vi "WS2812 Write N Pixels.vi"(7 "Refresh?":bool=TRUE, 8 "Error In":errorcluster, 9 "Colors":u32[](array[colorbox]), 10 "Start Pixel Index":u16, 11 "LINX Device Config":T1) -> (0 "Error Out":errorcluster, 3 "LINX Device Config":T1)   [LabVIEW 2014, in "LMH-LINX.lvlib" / "Device.lvlib"]
uses:
  <vilib>/MakerHub/LINX/Private/Device/Device.lvlib
  <vilib>/MakerHub/LINX/Private/Device/Type Defs/LINX Device Config.ctl
  <vilib>/MakerHub/LINX/Private/Type Defs/Interface.ctl
  <vilib>/MakerHub/LINX/Private/Device/Type Defs/TCP Config.ctl
  <vilib>/MakerHub/LINX/Private/Device/Type Defs/Channels.ctl
  <vilib>/MakerHub/LINX/Private/Type Defs/Error Type.ctl
  <vilib>/MakerHub/LINX/LMH-LINX.lvlib
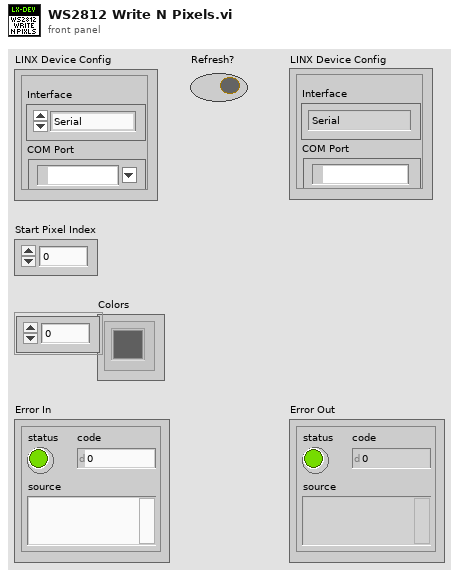
[diagram p1: front panel]
types:
  T1 = typedef "LMH-LINX.lvlib/Device.lvlib/LINX Device Config.ctl" = cluster{"Interface":T2, "COM Port":refnum<visa-resource-name>, "TCP Configuration":T3, "Device Family":u8, "Device ID":u8, "Device Name":string, "TCP Ref":refnum<k5>, "Channels":T4}
  T2 = typedef "LMH-LINX.lvlib/Interface.ctl" = enum16{"Serial", "TCP"}
  T3 = typedef "LMH-LINX.lvlib/Device.lvlib/TCP Config.ctl" = cluster{"IP Address":string, "Port":u16}
  T4 = typedef "LMH-LINX.lvlib/Channels.ctl" = cluster{"DI":u8[], "DO":u8[], "AI":u8[], "AO":u8[], "PWM":u8[], "QE":u8[], "UART":u8[], "I2C 2":u8[], "SPI":u8[], "CAN":u8[], "Servo":u8[], "AI Ref (V)":dbl, "AI Resolution (Bits)":u8, "AO Ref (V)":dbl, "AO Resolution (Bits)":u8}
  T5 = typedef "LMH-LINX.lvlib/Error Type.ctl" = enum16{"Unknown", "Timeout", "Corrupt Return Packet", "Unable To Connect", "Command Not Supported", "Channel DNE", "Invalid COM Config", "Firmware Version Mismatch", "myRIO Support", "CMD Specific Error", "Local IO Not Supported"}
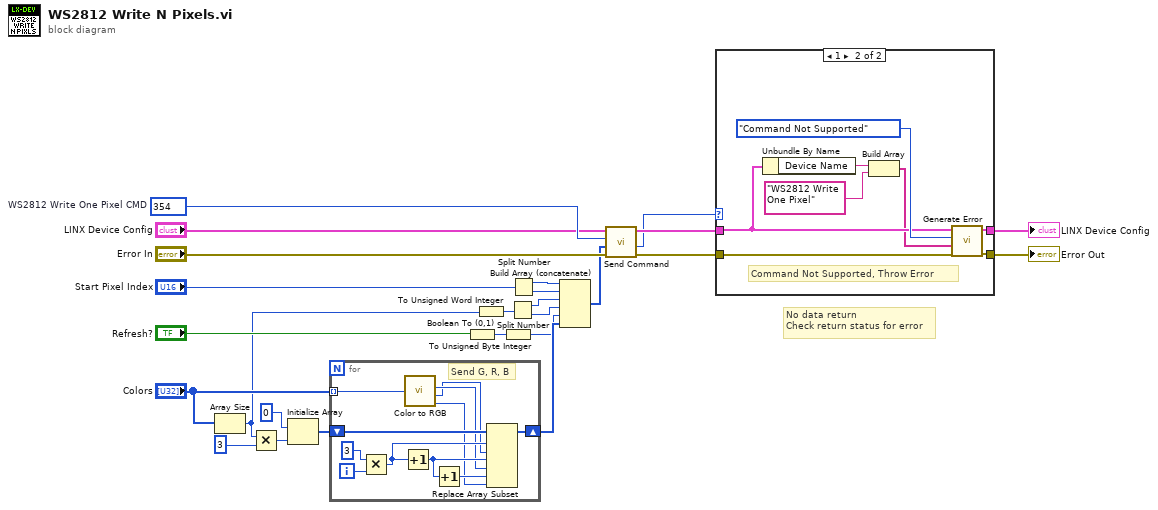
[diagram p0: block diagram]
diagram:
  w25 = u16 354  # WS2812 Write One Pixel CMD
  # "No data return\nCheck return status for error"
  n1 = Array Size(array="Colors") -> (size(s)=w1:i32)
  n2 = Multiply(x=w1, y=3) -> (x*y=w9:i32)
  n3 = Initialize Array(u8 0 ("y"), w9) -> (w7:u8[])
  n4 = for {
    tunnel: "Colors" -> [w36] mode=indexing
    shift-right: [w28] -> w6
    shift-left: w7 -> [w35]
    i -> [w33]
    # "Send G, R, B"
    n5 = Multiply(x=3 ("y"), y=w33) -> (x*y=w32:i32)
    n6 = Increment(x=w32) -> (x+1=w31:i32)
    n7 = call <vilib>:"Color to RGB.vi"("Color"=w36) -> ("R"=w27:u8, "G"=w26:u8, "B"=w29:u8)  [unwired: 1 out]
    n8 = Increment(x=w31) -> (x+1=w30:i32)
    n9 = Replace Array Subset(array=w35, new element #1=w26, index #1=w32, new element #2=w27, index #2=w31, new element #3=w29, index #3=w30) -> (w28:u8[])
  }
  n10 = Boolean To (0,1)(Boolean="Refresh?") -> (0, 1=w12:i16)
  n11 = To Unsigned Word Integer(number=w1) -> (unsigned 16bit integer=w2:u16)
  n12 = To Unsigned Byte Integer(number=w12) -> (unsigned 8bit integer=w5:u8)
  n13 = Split Number(x=w2) -> (hi(x)=w4:u8, lo(x)=w3:u8)
  n14 = Split Number(x="Start Pixel Index") -> (hi(x)=w16:u8, lo(x)=w15:u8)
  n15 = Build Array (concatenate)(w16, w15, w4, w3, w5, w6) -> (w14:u8[])
  n16 = call <vilib>:"Send Command.vi"("Error In"="Error In", "ARGS"=w14, "CMD"=w25, "LINX Device Config"="LINX Device Config") -> ("Error Out"=w22:errorcluster, "Status"=w20:u8, "LINX Device Config"=w21:T1)  [unwired: 4 in, 1 out]
  n17 = case shown="1" w20 {
    tunnel: [w38 w44] -> w24
    tunnel: w21 -> [w38 w40]
    tunnel: [w37 w45] -> w23
    tunnel: w22 -> [w37 w46]
    frame 0, Default {
      # "Status OK"
    }
    frame 1 {
      # "Command Not Supported, Throw Error"
      n18 = Unbundle By Name(w40) -> ("Device Name"=w42:string)
      n19 = Build Array(w42, "WS2812 Write One Pixel") -> (w39:string[])
      n20 = call <vilib>:"Generate Error.vi"("Error In"=w46, "Arguments"=w39, "Error Type"=Error_Type."Command Not Supported", "LINX Device Config"=w40) -> ("Error Out"=w45:errorcluster, "Dup LINX Device Config"=w44:T1)  [unwired: 6 in]
    }
  }
  "Error Out" <- w23
  "LINX Device Config" <- w24
